vi "AtSpectrograph_getEvent_loopTimeOutOfRange.vi"(8 "error in (no error)":errorcluster, 11 "logevent_loopTimeOutOfRange_Ctl":T1) -> (0 "error out":errorcluster, 2 "function return":i32, 3 "logevent_loopTimeOutOfRange_Ctl out":T1)   [LabVIEW 2016, in "SALLV_AtSpectrograph.lvlib"]
doc: "int AtSpectrograph_shm_getEvent_loopTimeOutOfRangeLV(AtSpectrograph_logevent_loopTimeOutOfRangeLV *logevent_loopTimeOutOfRange_Ctl );"
uses:
  SALLV_AtSpectrograph.lvlib
  DataTypes/logevent_loopTimeOutOfRange.ctl
  SALLV_AtSpectrograph.so
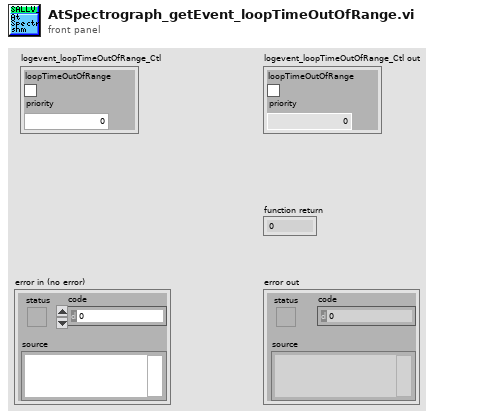
[diagram p1: front panel]
types:
  T1 = typedef "SALLV_AtSpectrograph.lvlib/logevent_loopTimeOutOfRange.ctl" = cluster{"loopTimeOutOfRange":bool, "priority":i32}
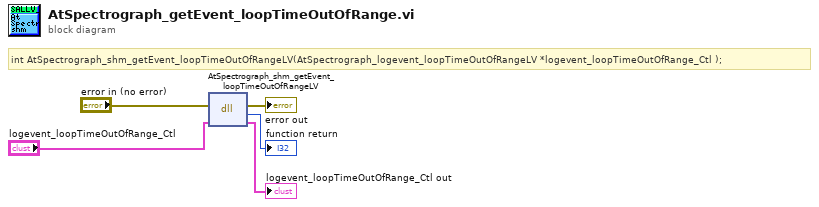
[diagram p0: block diagram]
diagram:
  # "int AtSpectrograph_shm_getEvent_loopTimeOutOfRangeLV(AtSpectrograph_logevent_loopTimeOutOfRangeLV *logevent_loopTimeOutOfRange_Ctl );"
  n1 = dll-call lib="home/harini/tcs/temp/SALLV_AtSpectrograph/SALLV_AtSpectrograph.*" fn="AtSpectrograph_shm_getEvent_loopTimeOutOfRangeLV"(error in="error in (no error)", "logevent_loopTimeOutOfRange_Ctl"="logevent_loopTimeOutOfRange_Ctl") -> (error out=→"error out":errorcluster, →"function return":i32, "logevent_loopTimeOutOfRange_Ctl"=→"logevent_loopTimeOutOfRange_Ctl out":T1)  [unwired: 2 in, 1 out]
